vi "Set SourceFile Path.vi"(8 "error in (no error)":errorcluster, 10 "SourceFile Path":path, 11 "ImageOperation in":refnum<class "ImageOperation.lvclass">) -> (0 "error out":errorcluster, 3 "ImageOperation out":refnum<class "ImageOperation.lvclass">)   [LabVIEW 2015, in "ImageOperation.lvclass"]
uses:
  ImageOperation.lvclass
  ImageOperation.lvclass/ImageOperation.ctl
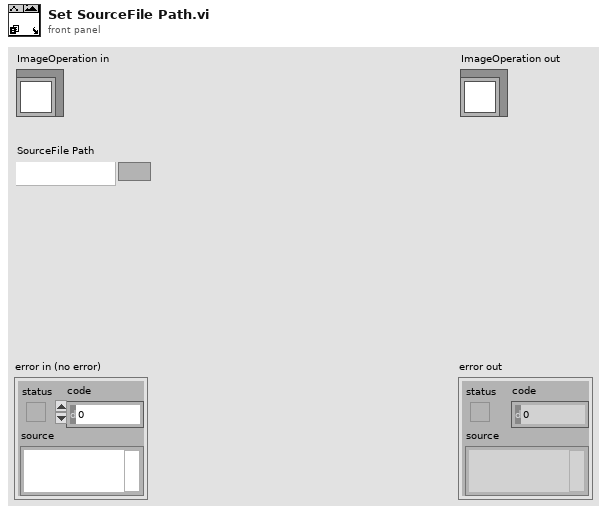
[diagram p1: front panel]
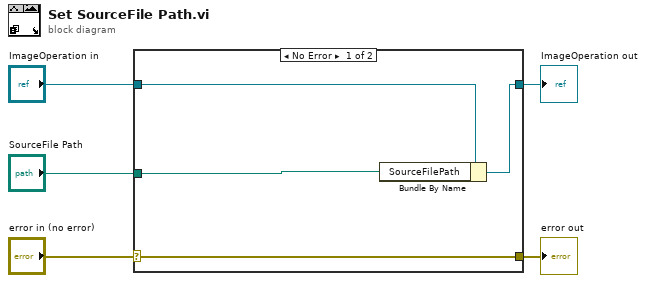
[diagram p0: block diagram]
diagram:
  n1 = case shown="No Error" "error in (no error)" {
    selector: "error in (no error)" -> [w9 w10]
    tunnel: [w9 w10] -> w4
    tunnel: [w7 w11] -> w2
    tunnel: "ImageOperation in" -> [w8 w11]
    tunnel: "SourceFile Path" -> [w6 _]
    frame No Error {
      n2 = Bundle By Name(cluster=w8, "SourceFilePath"=w6) -> (w7:refnum<class "ImageOperation.lvclass">)
    }
    frame Error {
    }
  }
  "error out" <- w4
  "ImageOperation out" <- w2
